vi "test.vi"() -> ()   [LabVIEW 2010]
uses:
  XMouseSlider.xctl
panel:
  in  "button:stop":bool
  in  "MouseSlider":dbl(xcontrol)
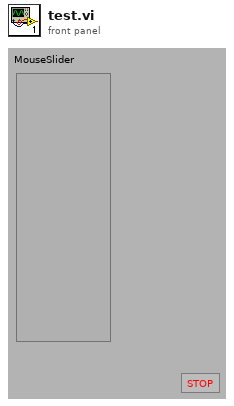
[diagram p1: front panel]
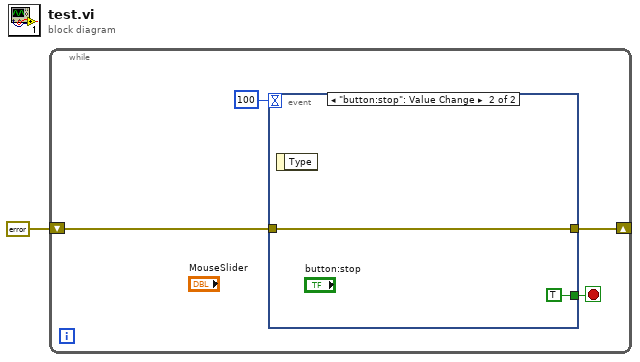
[diagram p0: block diagram]
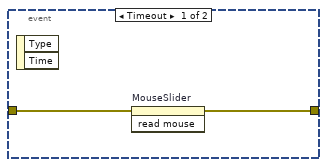
[diagram p2: hidden frame]
diagram:
  n1 = while {
    shift-right: [w3] -> _
    shift-left: errorcluster {"status"=FALSE, "code"=0, "source"=""} ("error in (no error)") -> [w4]
    stop <- w2 stop-if-true
    n2 = event shown="[1] \"button:stop\": Value Change" {
      selector: _ -> [_ _]
      dyn-events: _ -> [_ _]
      timeout: 100 -> [_ _]
      tunnel: w4 -> [w7 w9]
      tunnel: [w6 w9] -> w3
      tunnel: [_ TRUE] -> w2
      event Timeout {
        n3 = event-data() -> ()  [unwired: 1 in, 2 out]
        n4 = invoke on="MouseSlider" class="XMouseSlider (strict)" method="read mouse"(error in=w7) -> (error out=w6:errorcluster)  [unwired: 2 in, 2 out]
      }
      event "button:stop": Value Change {
        n5 = event-data() -> ()  [unwired: 1 in, 1 out]
      }
    }
  }
